vi "Zombie Left Cell.vi"(8 "Error In":errorcluster, 10 "Bookmark ID":u32, 11 "VI Info":T1) -> (0 "Error Out":errorcluster, 1 "Bold?":bool, 2 "Color":u32(colorbox)=40705, 3 "Text":string)   [LabVIEW 2018, in "Bookmark Manager.lvlib"]
doc: "Gets the left cell string for a zombie child item in the bookmarks tree. If the Spirit frame is enabled, then the text is \"Corpse\". If the Corpse frame is enabled, then the text is \"Reanimated\"."
uses:
  Bookmark Manager.lvlib
  Controls/VI Information.ctl
  Controls/Application Information.ctl
  Controls/Zombie States.ctl
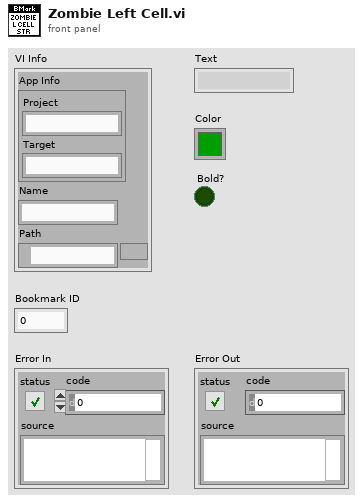
[diagram p1: front panel]
types:
  T1 = typedef "Bookmark Manager.lvlib/VI Information.ctl" = cluster{"App Info":T2, "Name":string, "Path":path}
  T2 = typedef "Bookmark Manager.lvlib/Application Information.ctl" = cluster{"Project":string, "Target":string}
  T3 = typedef "Bookmark Manager.lvlib/Zombie States.ctl" = enum16{"Corpse", "Reanimated"}
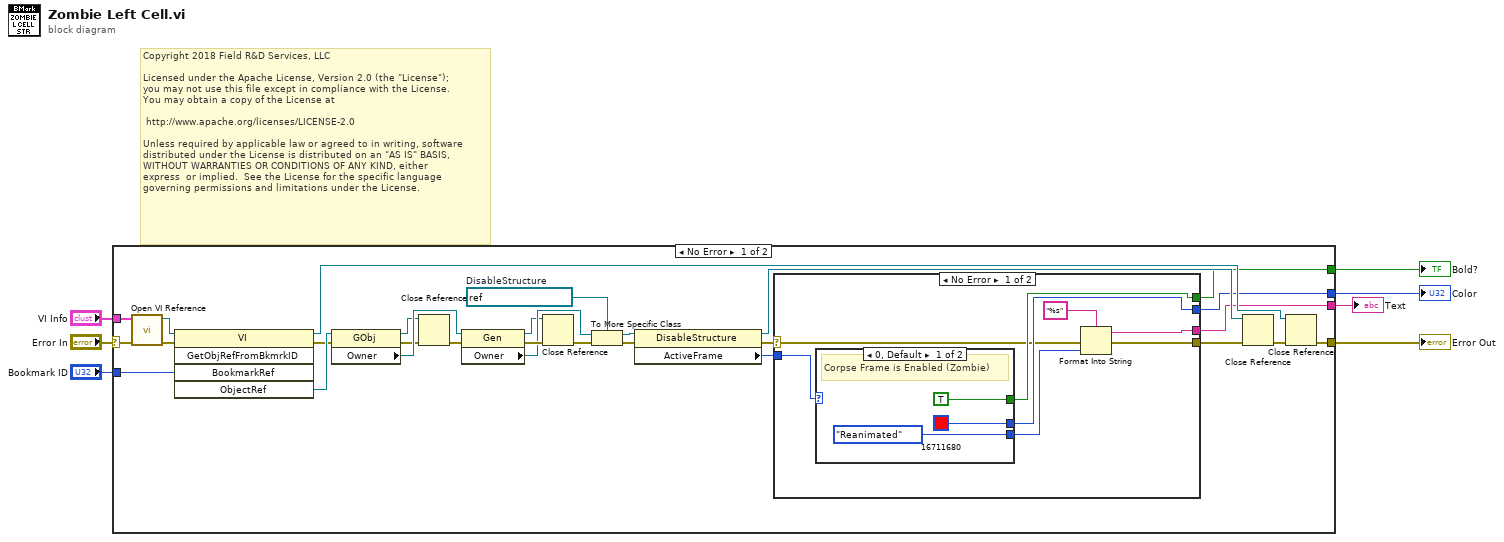
[diagram p0: block diagram]
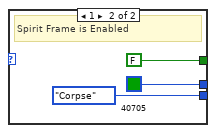
[diagram p2: hidden frame]
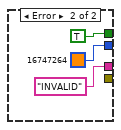
[diagram p3: hidden frame]
diagram:
  # "Copyright 2018 Field R&D Services, LLC\n\nLicensed under the Apache License, Version 2.0 (the \"License\");\nyou may not use this file except in compliance with the License.\nYou may obtain a copy of the License at\n\n\thttp://www.apache.org/licenses/LICENSE-2.0\n\nUnless required by applicable law or agreed to in writing, software\ndistributed under the License is distributed on an \"AS IS\" BASIS,\nWITHOUT WARRANTIES OR CONDITIONS OF ANY KIND, either \nexpress  or implied.  See the License for the specific language \ngoverning permissions and limitations under the License."
  n1 = case shown="No Error" "Error In" {
    selector: "Error In" -> [w14 w53]
    tunnel: "Bookmark ID" -> [w34 _]
    tunnel: [w12 w53] -> w6
    tunnel: [w17 _] -> w5
    tunnel: [w16 _] -> w4
    tunnel: [w15 _] -> w3
    tunnel: "VI Info" -> [w9 _]
    frame No Error {
      w33 = refnum<vi> refnum  # DisableStructure
      n2 = call "Open VI Reference.vi"("Error In"=w14, "VI Info"=w9) -> ("Error Out"=w10:errorcluster, "VI"=w8:refnum<vi>)  [unwired: 8 in]
      n3 = invoke class="VI" method="GetObjRefFromBkmrkID"(reference=w8, error in=w10, "BookmarkRef"=w34) -> (reference out=w27:refnum<vi>, error out=w18:errorcluster, "ObjectRef"=w35:refnum<vi>)  [unwired: 2 in, 2 out]
      n4 = property class="GObj"(reference=w35, error in=w18) -> (reference out=w24:refnum<vi>, error out=w25:errorcluster, "Owner"=w28:refnum<vi>)
      n5 = Close Reference(reference=w24, error in (no error)=w25) -> (error out=w23:errorcluster)
      n6 = property class="Gen"(reference=w28, error in=w23) -> (reference out=w19:refnum<vi>, error out=w22:errorcluster, "Owner"=w21:refnum<vi>)
      n7 = Close Reference(reference=w19, error in (no error)=w22) -> (error out=w20:errorcluster)
      n8 = To More Specific Class(target class=w33, reference=w21, error in=w20) -> (specific class reference=w32:refnum<vi>, error out=w31:errorcluster)
      n9 = property class="DisableStructure"(reference=w32, error in=w31) -> (reference out=w29:refnum<vi>, error out=w11:errorcluster, "ActiveFrame"=w30:i16)
      n10 = case shown="No Error" w11 {
        selector: w11 -> [w36 _]
        tunnel: w30 -> [w43 _]
        tunnel: [w40 "INVALID"] -> w17
        tunnel: [w39 TRUE] -> w16
        tunnel: [w38 u32 16747264] -> w15
        tunnel: [w37 _] -> w13
        frame No Error {
          n11 = case shown="0, Default" w43 {
            tunnel: [Zombie_States."Reanimated" ("Zombie State") Zombie_States."Corpse" ("Zombie State")] -> w42
            tunnel: [TRUE FALSE] -> w39
            tunnel: [u32 16711680 u32 40705] -> w38
            frame 0, Default {
              # "Corpse Frame is Enabled (Zombie)"
            }
            frame 1 {
              # "Spirit Frame is Enabled"
            }
          }
          n12 = Format Into String(format string="%s", error in=w36, w42) -> (resulting string=w40:string, error out=w37:errorcluster)  [unwired: 1 in]
        }
        frame Error {
        }
      }
      n13 = Close Reference(reference=w29, error in (no error)=w13) -> (error out=w26:errorcluster)
      n14 = Close Reference(reference=w27, error in (no error)=w26) -> (error out=w12:errorcluster)
    }
    frame Error {
    }
  }
  "Error Out" <- w6
  "Text" <- w5
  "Bold?" <- w4
  "Color" <- w3
